vi "mag_tear_down.vi"(8 "error in (no error)":errorcluster, 11 "magnetometer in":refnum<class "magnetometer.lvclass">) -> (0 "error out":errorcluster, 3 "magnetometer out":refnum<class "magnetometer.lvclass">)   [LabVIEW 2015, in "magnetometer.lvclass"]
uses:
  magnetometer.lvclass
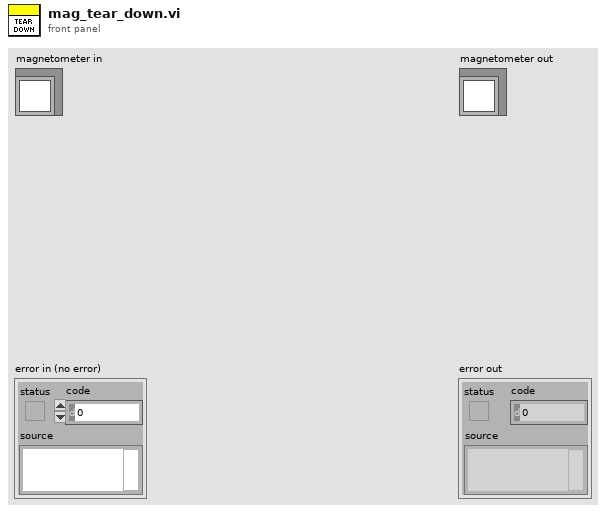
[diagram p1: front panel]
types:
  T1 = cluster{"input 1 task out":refnum<k21>, "input 2 task out":refnum<k21>}
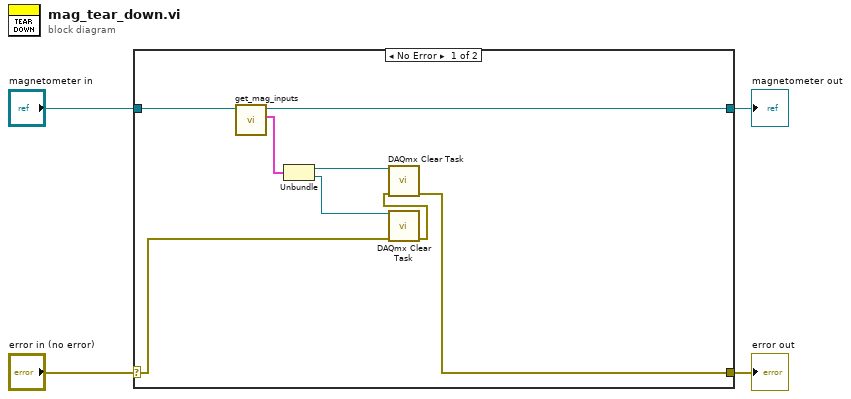
[diagram p0: block diagram]
diagram:
  n1 = case shown="No Error" "error in (no error)" {
    selector: "error in (no error)" -> [w7 w14]
    tunnel: [w5 w14] -> w3
    tunnel: [w11 w13] -> w1
    tunnel: "magnetometer in" -> [w12 w13]
    frame No Error {
      n2 = call-dynamic "get_mag_inputs.vi"("magnetometer in"=w12) -> ("mag inputs"=w10:T1, "magnetometer out"=w11:refnum<class "magnetometer.lvclass">)  [unwired: 8 in, 1 out]
      n3 = Unbundle(w10) -> ("input 1 task out"=w9:refnum<k21>, "input 2 task out"=w8:refnum<k21>)
      n4 = call <vilib>:"DAQmx Clear Task.vi"("task in"=w8, "error in"=w7) -> ("error out"=w6:errorcluster)  [unwired: 13 in]
      n5 = call <vilib>:"DAQmx Clear Task.vi"("task in"=w9, "error in"=w6) -> ("error out"=w5:errorcluster)  [unwired: 13 in]
    }
    frame Error {
    }
  }
  "error out" <- w3
  "magnetometer out" <- w1
